vi "GetIcon.vi"() -> ()   [LabVIEW 2014]
uses:
  <vilib>/Instr/_visa.llb/VISA Open Access Mode.ctl
panel:
  out "sortie d'erreur":errorcluster
  out "chaîne en sortie":string
  in  "Image to draw":i32
  out "spreadsheet string":string
  out "Array":u16[](array[numeric])
  # "TODO: envoyer le buffer d'image sur USB par blocs de 64 U8"
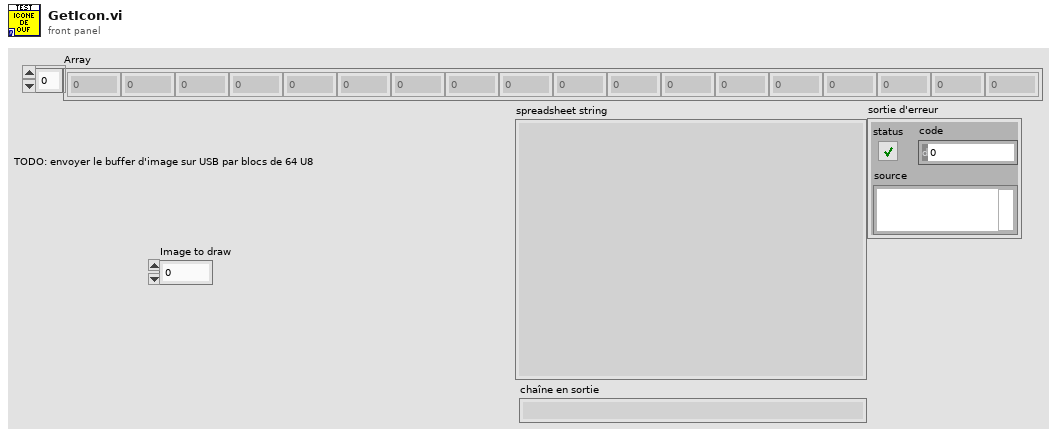
[diagram p1: front panel]
types:
  T1 = typedef "VISA Open Access Mode.ctl" = u32
  T2 = typedef "imagedata.ctl" = cluster{"image type":i32, "image depth":i32, "image":u8[], "mask":u8[], "colors":u32[], "Rectangle":cluster{"left":i16, "top":i16, "right":i16, "bottom":i16}}
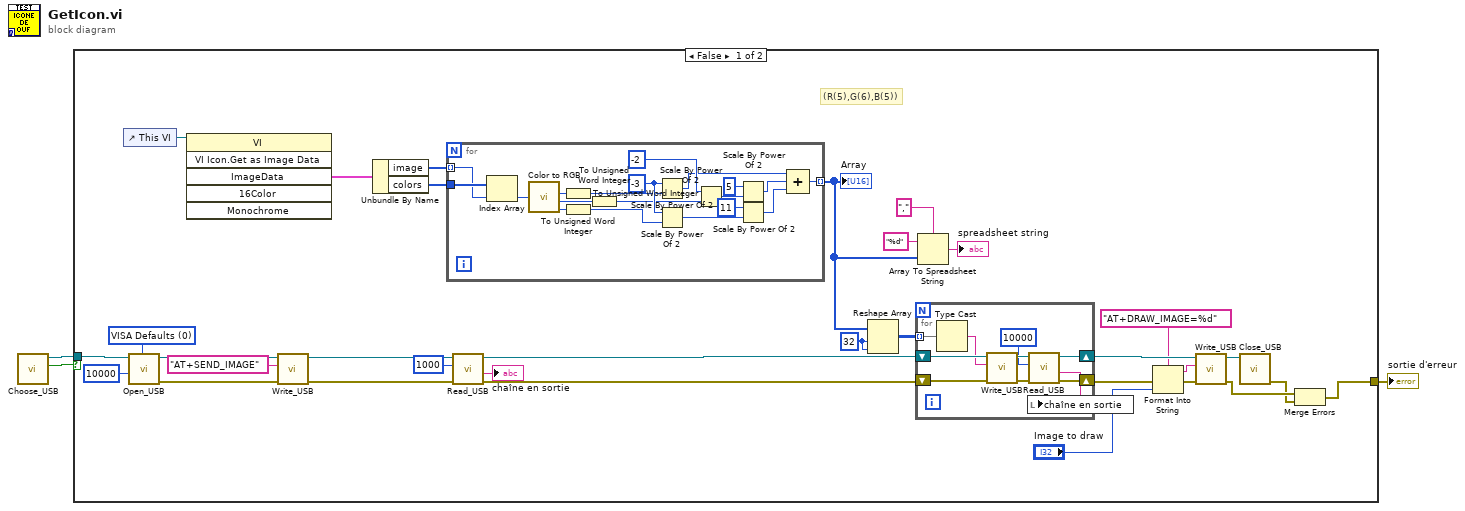
[diagram p0: block diagram]
diagram:
  n1 = call "Choose_USB.vi"() -> ("Annulé?"=w2:bool, "Nom de ressource VISA en sortie"=w3:refnum<visa-resource-name>)  [unwired: 10 in]
  n2 = case shown="False" w2 {
    tunnel: w3 -> [w28 _]
    tunnel: [w5 _] -> w1
    frame False {
      w4 = T1 0 items=["VISA Defaults"=0, "Exclusive Lock"=1, "Load Configured Settings"=4] ("Access Mode")
      w26 = 32 ("dimension size")
      # "(R(5),G(6),B(5))"
      n3 = control-ref of="This VI"() -> (w35:refnum<vi>)
      n4 = call "Open_USB.vi"("Timeout (0)"=u32 10000 ("Timeout de VISA Open (0)"), "Access Mode"=w4, "Nom de ressource VISA"=w28) -> ("error out"=w22:errorcluster, "Nom de ressource VISA ouverte"=w25:refnum<visa-resource-name>)  [unwired: 7 in]
      n5 = invoke class="VI" method="VI Icon.Get as Image Data"(reference=w35) -> ("ImageData"=w34:T2)  [unwired: 5 in, 5 out]
      n6 = call "Write_USB.vi"("entrée d'erreur"=w22, "buffer d'écriture"="AT+SEND_IMAGE", "Nom de ressource VISA"=w25) -> ("sortie d'erreur"=w12:errorcluster, "Nom de ressource VISA en sortie"=w14:refnum<visa-resource-name>)  [unwired: 7 in]
      n7 = Unbundle By Name(w34) -> ("image"=w33:u8[], "colors"=w32:u32[])
      n8 = for {
        tunnel: w33 -> [w63] mode=indexing
        tunnel: w32 -> [w64]
        tunnel: [w48] -> w27 mode=indexing
        w61 = i16 -3 ("n")
        n9 = Index Array(array=w64, index=w63) -> (element=w62:u32)
        n10 = call <vilib>:"Color to RGB.vi"("Color"=w62) -> ("R"=w57:u8, "G"=w56:u8, "B"=w54:u8)  [unwired: 1 out]
        n11 = To Unsigned Word Integer(number=w57) -> (unsigned 16bit integer=w46:u16)
        n12 = To Unsigned Word Integer(number=w54) -> (unsigned 16bit integer=w47:u16)
        n13 = To Unsigned Word Integer(number=w56) -> (unsigned 16bit integer=w55:u16)
        n14 = Scale By Power Of 2(n=w61, x=w46) -> (x*2^n=w51:u16)
        n15 = Scale By Power Of 2(n=w61, x=w47) -> (x*2^n=w53:u16)
        n16 = Scale By Power Of 2(n=i16 -2, x=w55) -> (x*2^n=w59:u16)
        n17 = Scale By Power Of 2(n=i16 5, x=w59) -> (x*2^n=w50:u16)
        n18 = Scale By Power Of 2(n=i16 11, x=w53) -> (x*2^n=w49:u16)
        n19 = Compound Arithmetic op=ADD(w51, w50, w49) -> (w48:u16)
      }
      "Array" <- w27
      n20 = call "Read_USB.vi"("entrée d'erreur"=w12, "timeout (0)"=u32 1000, "Nom de ressource VISA"=w14) -> ("sortie d'erreur"=w11:errorcluster, "chaîne en sortie"=→"chaîne en sortie":string, "Nom de ressource VISA en sortie"=w13:refnum<visa-resource-name>)  [unwired: 6 in]
      n21 = Reshape Array(w27, w26, w26) -> (w23:u16[][])
      n22 = for {
        tunnel: w23 -> [w44] mode=indexing
        shift-right: [w39] -> w20
        shift-left: w11 -> [w43]
        shift-right: [w41] -> w21
        shift-left: w13 -> [w45]
        n23 = Type Cast(x=w44) -> (*(type *) &x=w36:string)  [unwired: 1 in]
        n24 = call "Write_USB.vi"("entrée d'erreur"=w43, "buffer d'écriture"=w36, "Nom de ressource VISA"=w45) -> ("sortie d'erreur"=w40:errorcluster, "Nom de ressource VISA en sortie"=w42:refnum<visa-resource-name>)  [unwired: 7 in]
        n25 = call "Read_USB.vi"("entrée d'erreur"=w40, "timeout (0)"=u32 10000, "Nom de ressource VISA"=w42) -> ("sortie d'erreur"=w39:errorcluster, "chaîne en sortie"=w37:string, "Nom de ressource VISA en sortie"=w41:refnum<visa-resource-name>)  [unwired: 6 in]
        n26 = local write "chaîne en sortie"(w37) -> ()
      }
      n27 = Array To Spreadsheet String(delimiter (Tab)=",", array=w27, 3:"%d" ("format string")) -> (spreadsheet string=→"spreadsheet string":string)
      n28 = Format Into String(format string="AT+DRAW_IMAGE=%d", error in=w20, "Image to draw") -> (resulting string=w16:string, error out=w19:errorcluster)  [unwired: 1 in]
      n29 = call "Write_USB.vi"("entrée d'erreur"=w19, "buffer d'écriture"=w16, "Nom de ressource VISA"=w21) -> ("sortie d'erreur"=w7:errorcluster, "Nom de ressource VISA en sortie"=w15:refnum<visa-resource-name>)  [unwired: 7 in]
      n30 = call "Close_USB.vi"("Nom de ressource VISA"=w15) -> ("sortie d'erreur"=w6:errorcluster)  [unwired: 10 in]
      n31 = Merge Errors(w7, w6) -> (w5:errorcluster)
    }
    frame True {
    }
  }
  "sortie d'erreur" <- w1
